vi "Generate_Graphs.vi"(11 "Data (GT, Pred)":sgl[][](array[numeric])) -> (3 "Report":T1 {"R" format="%#_7g"})   [LabVIEW 2020]
uses:
  Controls/Regression_Report.ctl
  <vilib>/Analysis/6fits.llb/Curve Fitting Criteria.ctl
  <vilib>/Analysis/NI_AALPro.lvlib
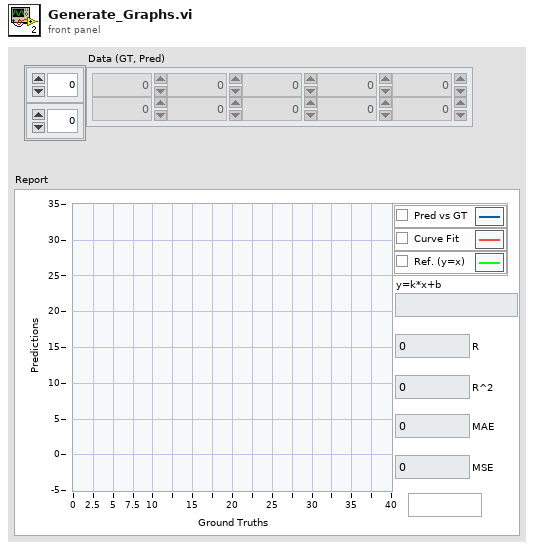
[diagram p1: front panel]
types:
  T1 = typedef "Regression_Report.ctl" = cluster{"Graphs":cluster{"Best Linear Fit":dbl[], "Array 3":sgl[]}[], "y=k*x+b":string, "R":sgl, "R^2":sgl, "MAE":sgl, "MSE":sgl}
  T2 = typedef "NI_AALPro.lvlib/Curve Fitting Criteria.ctl" = u16
  T3 = cluster{"Data (GT, Pred)":sgl[], "Data (GT, Pred)":sgl[]}
  T4 = cluster{"Best Linear Fit":dbl[], "Data (GT, Pred)":sgl[]}
  T5 = cluster{"Best Linear Fit":dbl[], "Data (GT, Pred)":sgl[]}[]
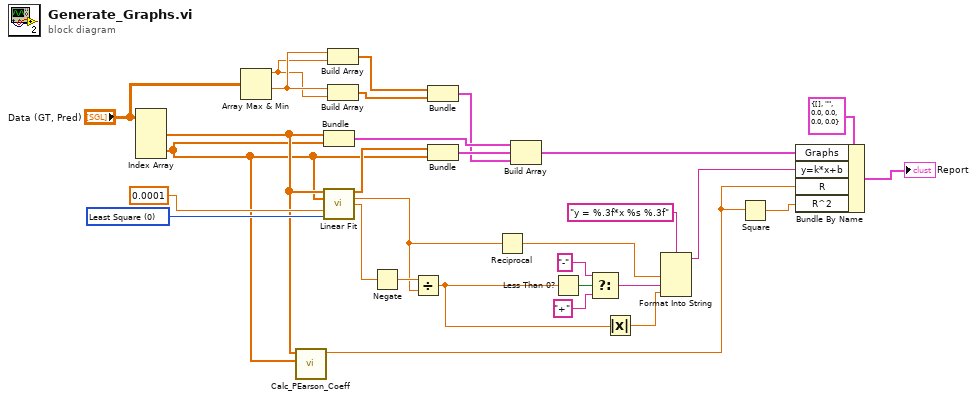
[diagram p0: block diagram]
diagram:
  w29 = T2 0 items=["Least Square", "Least Absolute Residual", "Bisquare"] ("method")
  n1 = Index Array(array="Data (GT, Pred)") -> (element #1=w8:sgl[], element #2=w7:sgl[])  [unwired: 4 in]
  n2 = Array Max & Min(array="Data (GT, Pred)") -> (max value=w20:sgl, min value=w21:sgl)  [unwired: 2 out]
  n3 = call "Calc_PEarson_Coeff.vi"("Y"=w7, "X"=w8) -> ("R"=w2:sgl)  [unwired: 9 in]
  n4 = Bundle("Data (GT, Pred)"=w8, "Data (GT, Pred)"=w7) -> (w30:T3)  [unwired: 1 in]
  n5 = call <vilib>:"Linear Fit.vi"("Y"=w8, "X"=w7, "tolerance"=0.0001, "method"=w29) -> ("Best Linear Fit"=w27:dbl[], "slope"=w9:dbl, "intercept"=w17:dbl)  [unwired: 7 in, 2 out]
  n6 = Build Array(w21, w20) -> (w24:sgl[])
  n7 = Build Array(w21, w20) -> (w23:sgl[])
  n8 = Negate(x=w17) -> (-x=w11:dbl)
  n9 = Divide(x=w11, y=w9) -> (x/y=w10:dbl)
  n10 = Bundle(w24, w23) -> (w22:cluster{sgl[], sgl[]})  [unwired: 1 in]
  n11 = Bundle("Best Linear Fit"=w27, "Data (GT, Pred)"=w7) -> (w26:T4)  [unwired: 1 in]
  n12 = Reciprocal(x=w9) -> (1/x=w12:dbl)
  n13 = Build Array(w30, w26, w22) -> (w4:T5)
  n14 = Less Than 0?(x=w10) -> (x < 0?=w16:bool)
  n15 = Select(t="-", s=w16, f="+") -> (s? t:f=w13:string)
  n16 = Absolute Value(x=w10) -> (abs(x)=w18:dbl)
  n17 = Format Into String(format string="y = %.3f*x %s %.3f", w12, w13, w18) -> (resulting string=w3:string)  [unwired: 2 in, 1 out]
  n18 = Square(x=w2) -> (x^2=w1:sgl)
  n19 = Bundle By Name(cluster=T1 {"Graphs"=[], "y=k*x+b"="", "R"=0.0, "R^2"=0.0, "MAE"=0.0, "MSE"=0.0} ("Report"), "Graphs"=w4, "y=k*x+b"=w3, "R"=w2, "R^2"=w1) -> (→"Report":T1)
